vi "analyze kHz maxcounts data.vi"(10 "Waveform Graph 3":sgl[](graph), 11 "ramp":i32[](array[numeric])) -> ()   [LabVIEW 2020]
uses:
  <userlib>/_OpenG.lib/array/array.llb/Index 1D Array Elements (SGL)__ogtk.vi
  <vilib>/Analysis/NI_AALPro.lvlib
panel:
  out "x-y":dbl[](array[numeric])
  out "peaks":cluster{dbl[], sgl[]}
  in  "Tab Control":T1(tab)=enum."1Hz peaks found"
  out "appended array":T2(graph)
  out "Locations":dbl[](array[numeric])
  out "Waveform Graph 4":sgl[](graph)
  out "Waveform Graph 5":sgl[](graph)
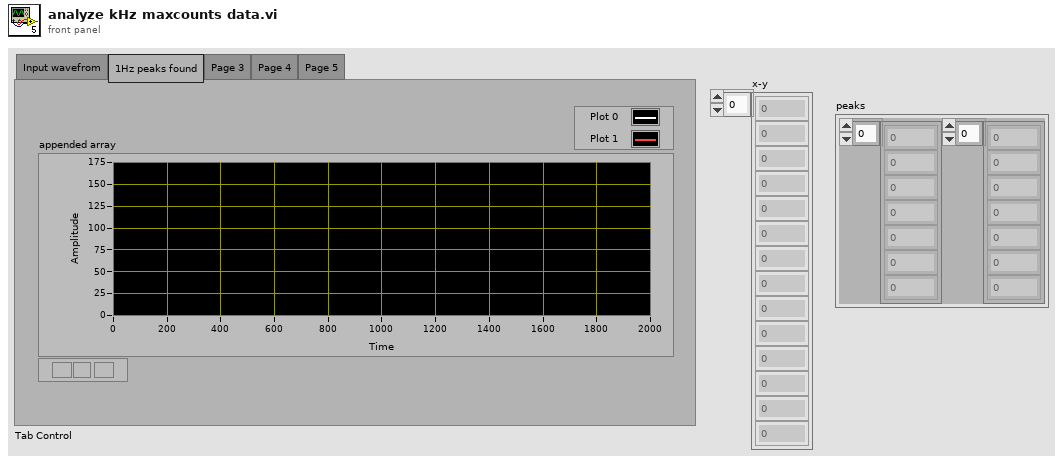
[diagram p1: front panel]
types:
  T1 = enum32{"Input wavefrom", "1Hz peaks found", "Page 3", "Page 4", "Page 5"}
  T2 = cluster{"ramp":i32[], "Waveform Graph 3":sgl[]}[]
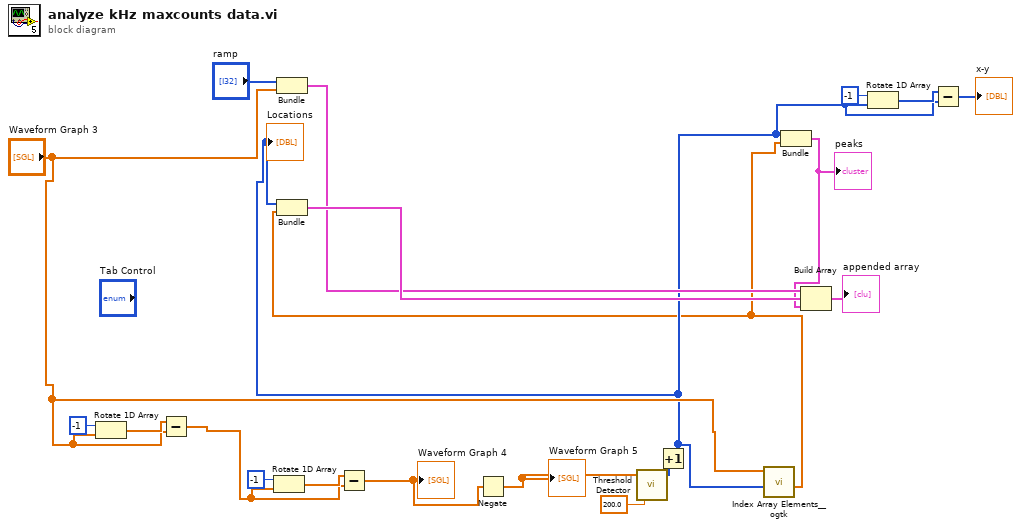
[diagram p0: block diagram]
diagram:
  n1 = Rotate 1D Array(1:"Waveform Graph 3", 2:-1 ("n")) -> (0:w12:sgl[])
  n2 = Subtract(x=w12, y="Waveform Graph 3") -> (x-y=w8:sgl[])
  n3 = Rotate 1D Array(1:w8, 2:-1 ("n")) -> (0:w10:sgl[])
  n4 = Bundle("ramp"="ramp", "Waveform Graph 3"="Waveform Graph 3") -> (w17:cluster{"ramp":i32[], "Waveform Graph 3":sgl[]})  [unwired: 1 in]
  n5 = Subtract(x=w10, y=w8) -> (x-y=w7:sgl[])
  "Waveform Graph 4" <- w7
  n6 = Negate(x=w7) -> (-x=w4:sgl[])
  "Waveform Graph 5" <- w4
  n7 = call <vilib>:"Threshold Detector.vi"("threshold"=200.0, "X"=w4) -> ("Indices"=w5:i32[])  [unwired: 1 in, 2 out]
  n8 = Increment(x=w5) -> (x+1=w2:i32[])
  "Locations" <- w2
  n9 = call-poly <userlib>:"Index Array Elements__ogtk.vi"("indices"=w2, "array"="Waveform Graph 3") -> ("elements"=w1:sgl[])  [unwired: 9 in]
  n10 = Bundle(w2, "elements"=w1) -> (w20:cluster{i32[], "elements":sgl[]})  [unwired: 1 in]
  n11 = Bundle(w2, "elements"=w1) -> (w16:cluster{i32[], "elements":sgl[]})  [unwired: 1 in]
  "peaks" <- w16
  n12 = Build Array(w17, w20, w16) -> (→"appended array":cluster{"ramp":i32[], "elements":sgl[]}[])
  n13 = Rotate 1D Array(1:w2, 2:-1 ("n")) -> (0:w15:i32[])
  n14 = Subtract(x=w15, y=w2) -> (x-y=→"x-y":i32[])
